vi "range_value.vi"() -> (2 "NumBins":i32, 3 "Center":i32)   [LabVIEW 2018]
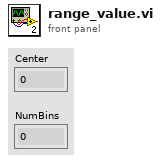
[diagram p1: front panel]
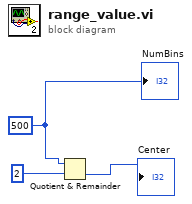
[diagram p0: block diagram]
diagram:
  w3 = 500
  n1 = Quotient & Remainder(x=w3, y=2) -> (floor(x/y)=→"Center":i32)  [unwired: 1 out]
  "NumBins" <- w3
